vi "setvelocity.vi"(8 "error in (no error)":errorcluster, 10 "Velocity":dbl, 11 "VISA in":refnum<visa-resource-name>) -> (0 "error out":errorcluster, 3 "VISA out":refnum<visa-resource-name>)   [LabVIEW 2015]
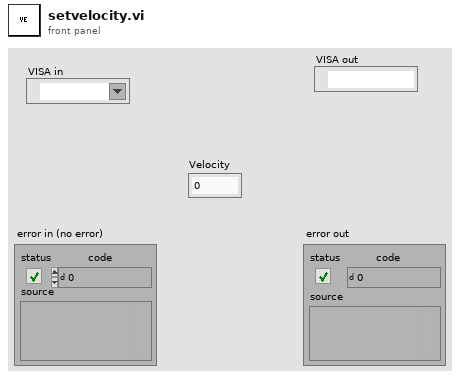
[diagram p1: front panel]
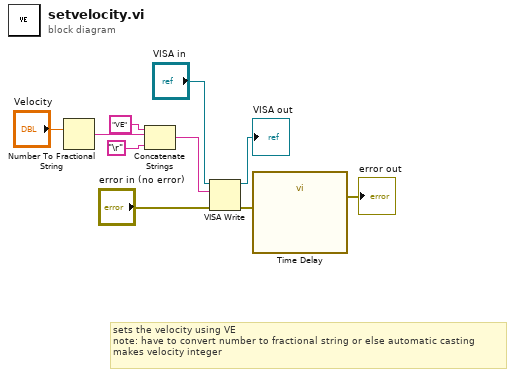
[diagram p0: block diagram]
diagram:
  # "sets the velocity using VE\nnote: have to convert number to fractional string or else automatic casting\nmakes velocity integer"
  n1 = Number To Fractional String(number="Velocity") -> (F-format string=w1:string)  [unwired: 3 in]
  n2 = Concatenate Strings("VE", w1, "\r") -> (w10:string)
  n3 = VISA Write(VISA resource name="VISA in", write buffer=w10, error in (no error)="error in (no error)") -> (VISA resource name out=→"VISA out":refnum<visa-resource-name>, error out=w4:errorcluster)  [unwired: 1 out]
  n4 = call "Time Delay"("error in (no error)"=w4) -> ("error out"=→"error out":errorcluster)  [unwired: 10 in]
